vi "MovePickPlace_org.vi"() -> ()   [LabVIEW 2019]
panel:
  in  "GoToZero":bool=TRUE
  in  "MoveToToolDropPosition":bool=TRUE
  in  "DropTool":bool=TRUE
  in  "DropPlate":bool=TRUE
  in  "MoveToAssemblyPosition":bool=TRUE
  in  "PickPlate":bool=TRUE
  in  "MoveToPlatePosition":bool=TRUE
  in  "PickTool":bool=TRUE
  in  "MoveToToolPosition":bool=TRUE
  out "Final":string
  in  "Move Z first 5":bool=TRUE
  in  "Absolute 5":bool=TRUE
  in  "SpeedZ (mm/s) 5":dbl=10.0
  in  "SpeedXY (mm/s) 5":dbl=100.0
  in  "Z 5":dbl
  in  "Y 5":dbl
  in  "X 5":dbl
  out "sensor on? 4":bool
  out "Tool Position drop":string
  in  "Move Z first 4":bool
  in  "Absolute 4":bool=TRUE
  in  "SpeedZ (mm/s) 4":dbl=10.0
  in  "SpeedXY (mm/s) 4":dbl=100.0
  in  "Z 4":dbl
  in  "Y 4":dbl=876.324
  in  "X 4":dbl=549.248
  out "sensor on? 3":bool
  out "Assembly Position":string
  in  "Move Z first 3":bool
  in  "Absolute 3":bool=TRUE
  in  "SpeedZ (mm/s) 3":dbl=10.0
  in  "SpeedXY (mm/s) 3":dbl=100.0
  in  "Z 3":dbl
  in  "Y 3":dbl=882.7703
  in  "X 3":dbl=250.9431
  out "sensor on? 2":bool
  out "sensor on?":bool
  out "error out":errorcluster
  out "Plate Position":string
  in  "Move Z first 2":bool
  in  "Absolute 2":bool=TRUE
  in  "SpeedZ (mm/s) 2":dbl=10.0
  in  "SpeedXY (mm/s) 2":dbl=100.0
  in  "Z 2":dbl
  in  "Y 2":dbl=876.2095
  in  "X 2":dbl=1126.3618
  out "Tool Position":string
  in  "Move Z first":bool
  in  "Absolute":bool=TRUE
  in  "SpeedZ (mm/s)":dbl=10.0
  in  "SpeedXY (mm/s)":dbl=100.0
  in  "Z":dbl
  in  "Y":dbl=876.3244
  in  "X":dbl=549.2477
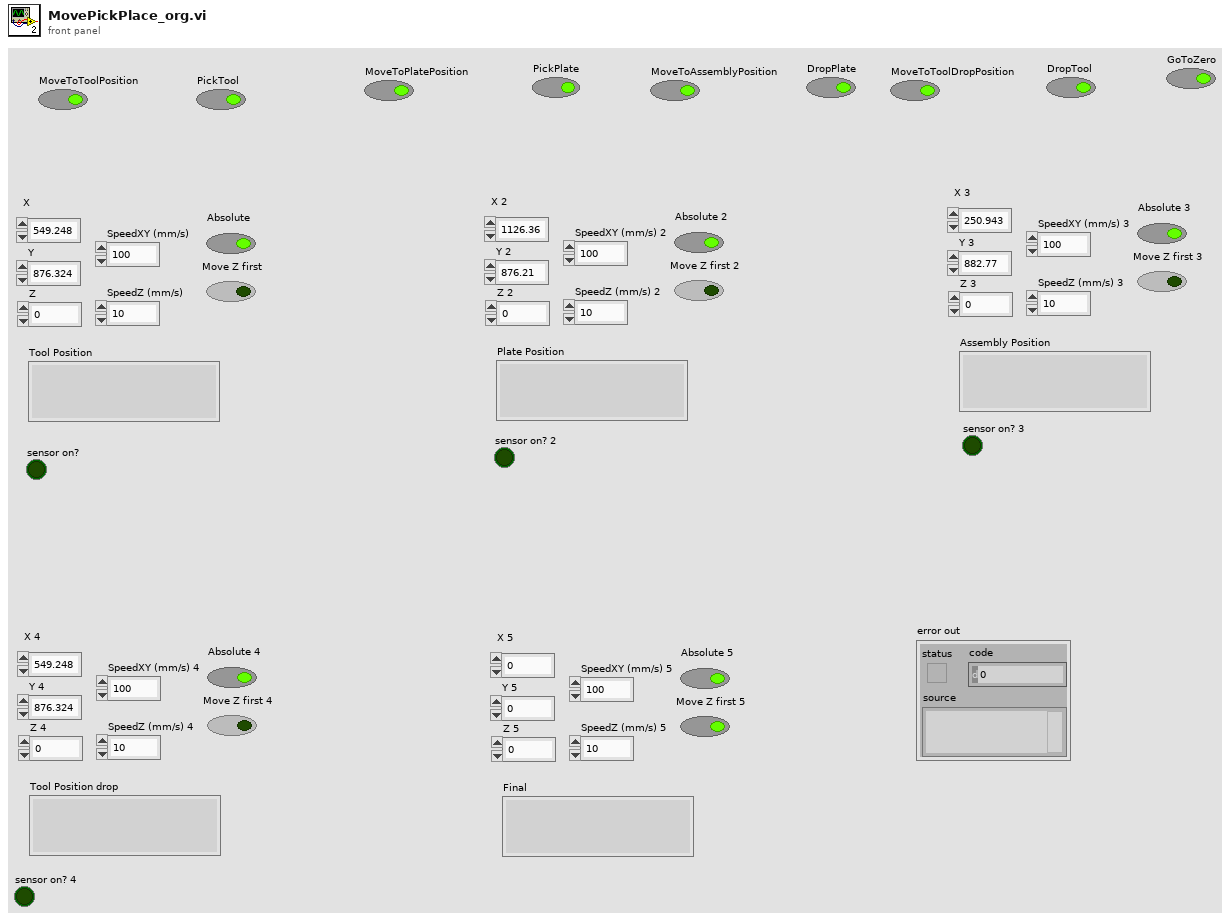
[diagram p1: front panel]
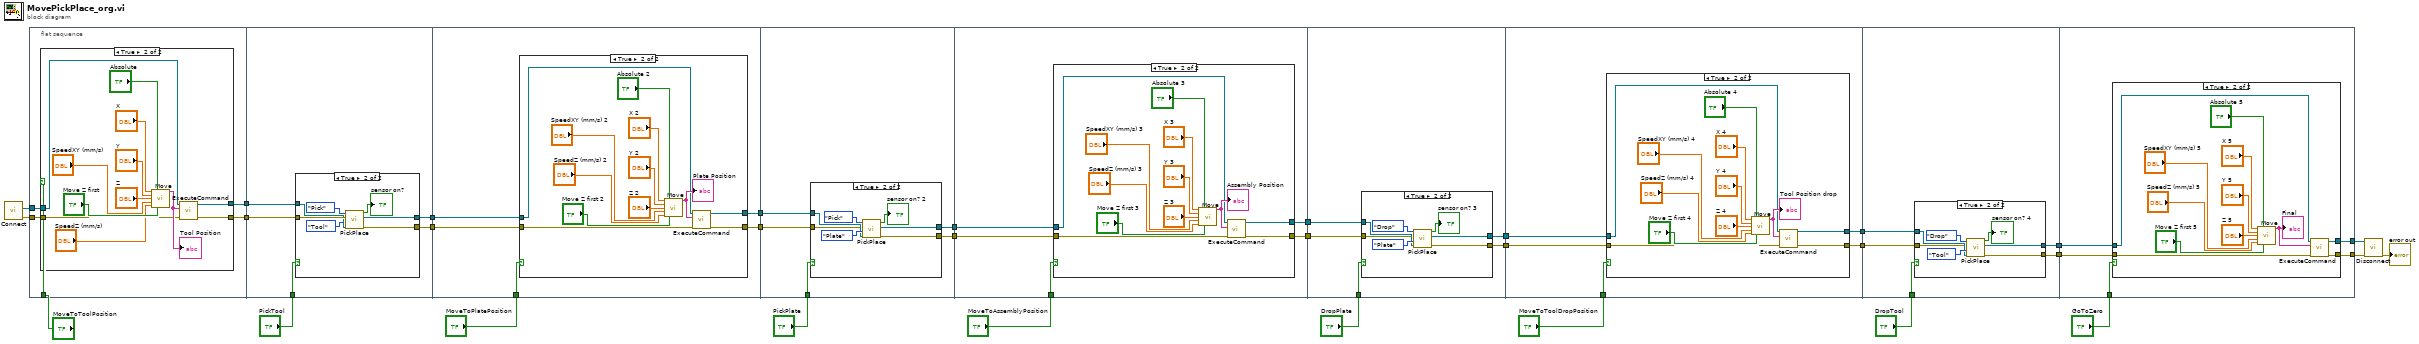
[diagram p0: block diagram]
diagram:
  n1 = call "Connect.vi"() -> ("error out"=w28:errorcluster, "controller"=w29:refnum<k24>)  [unwired: 10 in]
  n2 = flat-sequence {
    tunnel: [w33] -> w25
    tunnel: w29 -> [w35]
    tunnel: w28 -> [w34]
    tunnel: [w32] -> w23
    tunnel: "MoveToToolPosition" -> [w31]
    tunnel: w25 -> [w54]
    tunnel: [w51] -> w24
    tunnel: w23 -> [w53]
    tunnel: [w52] -> w22
    tunnel: "PickTool" -> [w50]
    tunnel: w24 -> [w67]
    tunnel: w22 -> [w68]
    tunnel: [w66] -> w21
    tunnel: [w65] -> w20
    tunnel: "MoveToPlatePosition" -> [w64]
    tunnel: w21 -> [w86]
    tunnel: w20 -> [w87]
    tunnel: [w84] -> w19
    tunnel: [w85] -> w18
    tunnel: "PickPlate" -> [w83]
    tunnel: w19 -> [w100]
    tunnel: w18 -> [w101]
    tunnel: [w99] -> w17
    tunnel: [w98] -> w16
    tunnel: "MoveToAssemblyPosition" -> [w97]
    tunnel: w17 -> [w117]
    tunnel: w16 -> [w119]
    tunnel: [w118] -> w15
    tunnel: [w120] -> w14
    tunnel: "DropPlate" -> [w116]
    tunnel: w15 -> [w133]
    tunnel: w14 -> [w134]
    tunnel: [w131] -> w13
    tunnel: [w132] -> w12
    tunnel: "MoveToToolDropPosition" -> [w130]
    tunnel: w13 -> [w152]
    tunnel: w12 -> [w153]
    tunnel: [w151] -> w11
    tunnel: [w150] -> w10
    tunnel: "DropTool" -> [w149]
    tunnel: [w165] -> w26
    tunnel: [w164] -> w27
    tunnel: w11 -> [w166]
    tunnel: w10 -> [w167]
    tunnel: "GoToZero" -> [w163]
    frame #0 {
      n3 = case shown="True" w31 {
        tunnel: w35 -> [w37 w41]
        tunnel: w34 -> [w36 w40]
        tunnel: [w36 w39] -> w33
        tunnel: [w37 w38] -> w32
        frame False {
        }
        frame True {
          n4 = call "Move.vi"("X"="X", "Absolute"="Absolute", "Y"="Y", "Z"="Z", "SpeedXY (mm/s)"="SpeedXY (mm/s)", "SpeedZ (mm/s)"="SpeedZ (mm/s)", "Move Z first"="Move Z first") -> ("Position Gcode"=w42:string)  [unwired: 8 in]
          "Tool Position" <- w42
          n5 = call "ExecuteCommand.vi"("error in (no error)"=w40, "Command Code"=w42, "controller in"=w41) -> ("error out"=w39:errorcluster, "controller out"=w38:refnum<k24>)  [unwired: 6 in, 1 out]
        }
      }
    }
    frame #1 {
      n6 = case shown="True" w50 {
        tunnel: w54 -> [w56 w62]
        tunnel: w53 -> [w55 w61]
        tunnel: [w55 w58] -> w52
        tunnel: [w56 w57] -> w51
        frame False {
        }
        frame True {
          n7 = call "PickPlace.vi"("controller"=w61, "Tool or Plate"=enum16{"Tool", "Plate"}."Tool", "error in (no error)"=w62, "Pick or Drop"=enum16{"Pick", "Drop"}."Pick") -> ("error out"=w57:errorcluster, "controller out"=w58:refnum<k24>, "sensor on?"=→"sensor on?":bool)  [unwired: 1 in]
        }
      }
    }
    frame #2 {
      n8 = case shown="True" w64 {
        tunnel: w68 -> [w69 w74]
        tunnel: w67 -> [w70 w73]
        tunnel: [w70 w72] -> w66
        tunnel: [w69 w71] -> w65
        frame False {
        }
        frame True {
          n9 = call "Move.vi"("X"="X 2", "Absolute"="Absolute 2", "Y"="Y 2", "Z"="Z 2", "SpeedXY (mm/s)"="SpeedXY (mm/s) 2", "SpeedZ (mm/s)"="SpeedZ (mm/s) 2", "Move Z first"="Move Z first 2") -> ("Position Gcode"=w75:string)  [unwired: 8 in]
          "Plate Position" <- w75
          n10 = call "ExecuteCommand.vi"("error in (no error)"=w73, "Command Code"=w75, "controller in"=w74) -> ("error out"=w72:errorcluster, "controller out"=w71:refnum<k24>)  [unwired: 6 in, 1 out]
        }
      }
    }
    frame #3 {
      n11 = case shown="True" w83 {
        tunnel: w87 -> [w88 w93]
        tunnel: w86 -> [w89 w92]
        tunnel: [w88 w91] -> w85
        tunnel: [w89 w90] -> w84
        frame False {
        }
        frame True {
          n12 = call "PickPlace.vi"("controller"=w93, "Tool or Plate"=enum16{"Tool", "Plate"}."Plate", "error in (no error)"=w92, "Pick or Drop"=enum16{"Pick", "Drop"}."Pick") -> ("error out"=w90:errorcluster, "controller out"=w91:refnum<k24>, "sensor on?"=→"sensor on? 2":bool)  [unwired: 1 in]
        }
      }
    }
    frame #4 {
      n13 = case shown="True" w97 {
        tunnel: w101 -> [w103 w107]
        tunnel: w100 -> [w102 w106]
        tunnel: [w102 w105] -> w99
        tunnel: [w103 w104] -> w98
        frame False {
        }
        frame True {
          n14 = call "Move.vi"("X"="X 3", "Absolute"="Absolute 3", "Y"="Y 3", "Z"="Z 3", "SpeedXY (mm/s)"="SpeedXY (mm/s) 3", "SpeedZ (mm/s)"="SpeedZ (mm/s) 3", "Move Z first"="Move Z first 3") -> ("Position Gcode"=w108:string)  [unwired: 8 in]
          "Assembly Position" <- w108
          n15 = call "ExecuteCommand.vi"("error in (no error)"=w106, "Command Code"=w108, "controller in"=w107) -> ("error out"=w105:errorcluster, "controller out"=w104:refnum<k24>)  [unwired: 6 in, 1 out]
        }
      }
    }
    frame #5 {
      n16 = case shown="True" w116 {
        tunnel: [w121 w126] -> w120
        tunnel: w119 -> [w121 w125]
        tunnel: [w122 w124] -> w118
        tunnel: w117 -> [w122 w123]
        frame False {
        }
        frame True {
          n17 = call "PickPlace.vi"("controller"=w125, "Tool or Plate"=enum16{"Tool", "Plate"}."Plate", "error in (no error)"=w123, "Pick or Drop"=enum16{"Pick", "Drop"}."Drop") -> ("error out"=w124:errorcluster, "controller out"=w126:refnum<k24>, "sensor on?"=→"sensor on? 3":bool)  [unwired: 1 in]
        }
      }
    }
    frame #6 {
      n18 = case shown="True" w130 {
        tunnel: w134 -> [w135 w140]
        tunnel: w133 -> [w136 w139]
        tunnel: [w135 w138] -> w132
        tunnel: [w136 w137] -> w131
        frame False {
        }
        frame True {
          n19 = call "Move.vi"("X"="X 4", "Absolute"="Absolute 4", "Y"="Y 4", "Z"="Z 4", "SpeedXY (mm/s)"="SpeedXY (mm/s) 4", "SpeedZ (mm/s)"="SpeedZ (mm/s) 4", "Move Z first"="Move Z first 4") -> ("Position Gcode"=w141:string)  [unwired: 8 in]
          "Tool Position drop" <- w141
          n20 = call "ExecuteCommand.vi"("error in (no error)"=w139, "Command Code"=w141, "controller in"=w140) -> ("error out"=w137:errorcluster, "controller out"=w138:refnum<k24>)  [unwired: 6 in, 1 out]
        }
      }
    }
    frame #7 {
      n21 = case shown="True" w149 {
        tunnel: w153 -> [w154 w159]
        tunnel: w152 -> [w155 w158]
        tunnel: [w155 w157] -> w151
        tunnel: [w154 w156] -> w150
        frame False {
        }
        frame True {
          n22 = call "PickPlace.vi"("controller"=w159, "Tool or Plate"=enum16{"Tool", "Plate"}."Tool", "error in (no error)"=w158, "Pick or Drop"=enum16{"Pick", "Drop"}."Drop") -> ("error out"=w157:errorcluster, "controller out"=w156:refnum<k24>, "sensor on?"=→"sensor on? 4":bool)  [unwired: 1 in]
        }
      }
    }
    frame #8 {
      n23 = case shown="True" w163 {
        tunnel: w167 -> [w168 w173]
        tunnel: w166 -> [w169 w172]
        tunnel: [w168 w171] -> w165
        tunnel: [w169 w170] -> w164
        frame False {
        }
        frame True {
          n24 = call "Move.vi"("X"="X 5", "Absolute"="Absolute 5", "Y"="Y 5", "Z"="Z 5", "SpeedXY (mm/s)"="SpeedXY (mm/s) 5", "SpeedZ (mm/s)"="SpeedZ (mm/s) 5", "Move Z first"="Move Z first 5") -> ("Position Gcode"=w174:string)  [unwired: 8 in]
          "Final" <- w174
          n25 = call "ExecuteCommand.vi"("error in (no error)"=w172, "Command Code"=w174, "controller in"=w173) -> ("error out"=w170:errorcluster, "controller out"=w171:refnum<k24>)  [unwired: 6 in, 1 out]
        }
      }
    }
  }
  n26 = call "Disconnect.vi"("error in (no error)"=w27, "controller"=w26) -> ("error out"=→"error out":errorcluster)  [unwired: 9 in]
